vi "Initialize SLSC Module.vi"(8 "error in (no error)":errorcluster, 9 "SLSC Custom Device Information":T1 {"Custom Device Information"."Driver VIs"."Supported Target" items=["All", "Pharlap", "VxWorks", "Windows", "Linux_32_ARM", "Linux_x64", "PharlapWindows", "PharlapVxWorks", "VxWorksWindows"]; "Custom Device Information"."Driver VIs"."Type" items=["Absolute", "ToBase", "ToCommonDocDir", "ToApplicationDataDir"]; "Custom Device Information"."Execution Mode" items=["Asynchronous", "InlineHWInterface", "InlineModelInterface", "InlineTimingandSync", "AsynchronousTimingandSync"]}, 10 "Name":string, 11 "SLSC Module":u64) -> (0 "error out":errorcluster, 3 "SLSC Module out":u64)   [LabVIEW 2017, in "VeriStand SLSC Scripting.lvlib"]
uses:
  VeriStand SLSC Scripting.lvlib
  Controls/SLSC Custom Device Information.ctl
  Controls/Custom Device Information.ctl
  Controls/Driver VI Information.ctl
  NationalInstruments.VeriStand.SystemDefinitionAPI
  NationalInstruments.VeriStand.SystemStorage
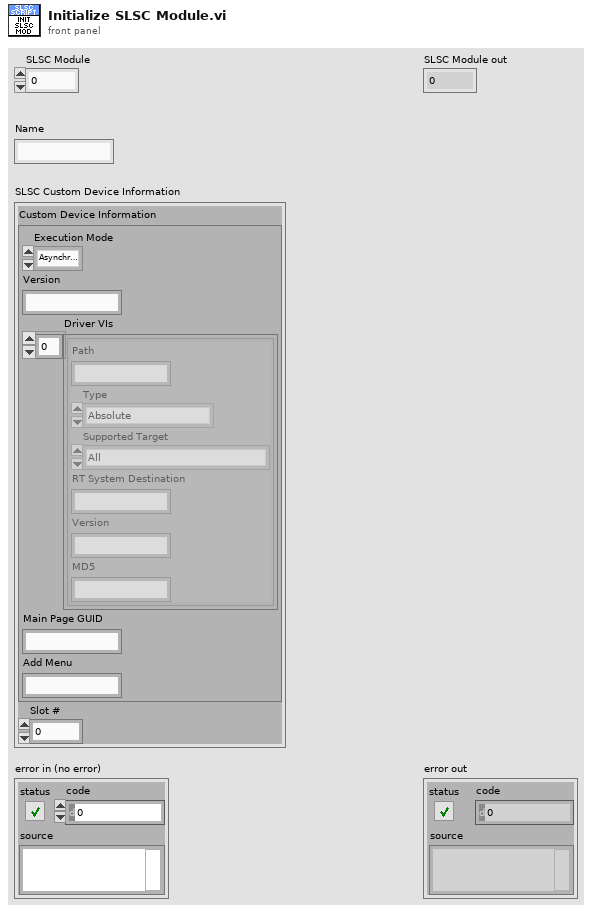
[diagram p1: front panel]
types:
  T1 = typedef "VeriStand SLSC Scripting.lvlib/SLSC Custom Device Information.ctl" = cluster{"Custom Device Information":T2, "Slot #":i32}
  T2 = typedef "VeriStand SLSC Scripting.lvlib/Custom Device Information.ctl" = cluster{"Execution Mode":i32, "Version":string, "Driver VIs":T3[], "Main Page GUID":string, "Add Menu":string}
  T3 = typedef "VeriStand SLSC Scripting.lvlib/Driver VI Information.ctl" = cluster{"Path":string, "Type":i32, "Supported Target":i32, "RT System Destination":string, "Version":string, "MD5":string}
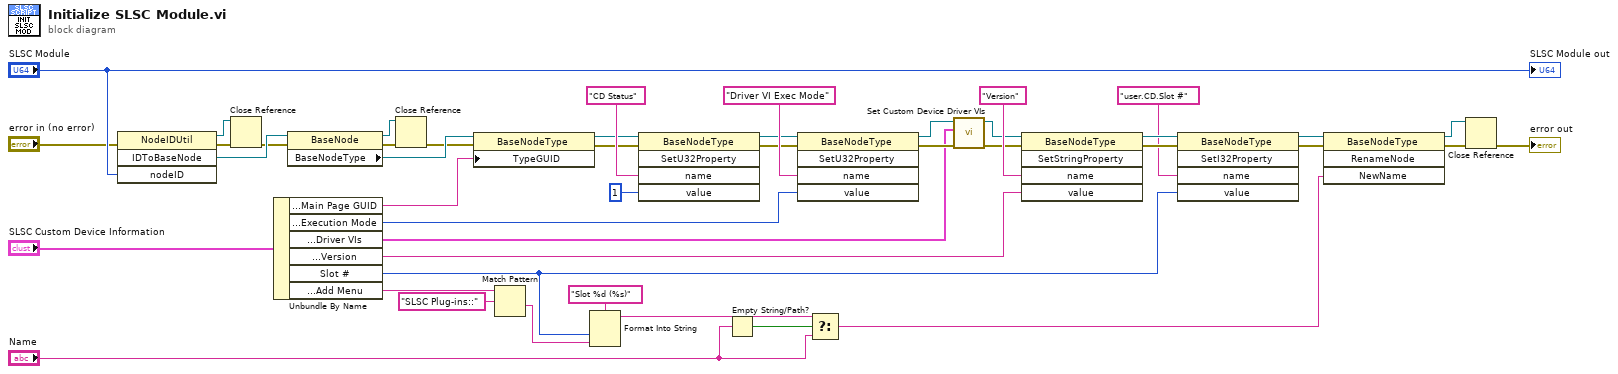
[diagram p0: block diagram]
diagram:
  n1 = invoke class="NodeIDUtil" method="IDToBaseNode"(error in="error in (no error)", "nodeID"="SLSC Module") -> (reference out=w19:refnum<k24>, error out=w21:errorcluster, "IDToBaseNode"=w15:refnum<k24>)  [unwired: 2 in, 1 out]
  n2 = Close Reference(reference=w19, error in (no error)=w21) -> (error out=w14:errorcluster)
  n3 = Unbundle By Name("SLSC Custom Device Information") -> ("Custom Device Information.Main Page GUID"=w42:string, "Custom Device Information.Execution Mode"=w34:i32, "Custom Device Information.Driver VIs"=w31:T3[], "Custom Device Information.Version"=w24:string, "Slot #"=w8:i32, "Custom Device Information.Add Menu"=w3:string)
  n4 = property class="BaseNode"(reference=w15, error in=w14) -> (reference out=w20:refnum<k24>, error out=w44:errorcluster, "BaseNodeType"=w17:refnum<k24>)
  n5 = Close Reference(reference=w20, error in (no error)=w44) -> (error out=w16:errorcluster)
  n6 = property class="BaseNodeType"(reference=w17, error in=w16, "TypeGUID"=w42) -> (reference out=w35:refnum<k24>, error out=w36:errorcluster)
  n7 = Match Pattern(string=w3, regular expression="SLSC Plug-ins::") -> (after substring=w1:string)  [unwired: 1 in, 3 out]
  n8 = Format Into String(format string="Slot %d (%s)", w8, w1) -> (resulting string=w5:string)  [unwired: 2 in, 1 out]
  n9 = invoke class="BaseNodeType" method="SetU32Property"(reference=w35, error in=w36, "name"="CD Status", "value"=u32 1) -> (reference out=w37:refnum<k24>, error out=w38:errorcluster)  [unwired: 1 in, 3 out]
  n10 = Empty String/Path?(string/path="Name") -> (empty?=w7:bool)
  n11 = invoke class="BaseNodeType" method="SetU32Property"(reference=w37, error in=w38, "name"="Driver VI Exec Mode", "value"=w34) -> (reference out=w32:refnum<k24>, error out=w33:errorcluster)  [unwired: 1 in, 3 out]
  n12 = Select(t=w5, s=w7, f="Name") -> (s? t:f=w4:string)
  n13 = call "Set Custom Device Driver VIs.vi"("error in (no error)"=w33, "Driver VIs"=w31, "BaseNodeType"=w32) -> ("error out"=w26:errorcluster, "BaseNodeType out"=w25:refnum<k24>)  [unwired: 7 in]
  n14 = invoke class="BaseNodeType" method="SetStringProperty"(reference=w25, error in=w26, "name"="Version", "value"=w24) -> (reference out=w28:refnum<k24>, error out=w29:errorcluster)  [unwired: 1 in, 3 out]
  n15 = invoke class="BaseNodeType" method="SetI32Property"(reference=w28, error in=w29, "name"="user.CD.Slot #", "value"=w8) -> (reference out=w12:refnum<k24>, error out=w13:errorcluster)  [unwired: 1 in, 3 out]
  n16 = invoke class="BaseNodeType" method="RenameNode"(reference=w12, error in=w13, "NewName"=w4) -> (reference out=w10:refnum<k24>, error out=w11:errorcluster)  [unwired: 1 in, 2 out]
  n17 = Close Reference(reference=w10, error in (no error)=w11) -> (error out=→"error out":errorcluster)
  "SLSC Module out" <- "SLSC Module"
